vi "Fetch Multi Eval Meas List ACLR Detected Allocation Results.vi"(8 "error in (no error)":errorcluster, 10 "Instance (1)":T2=1, 11 "VISA resource name":refnum<visa-resource-name>) -> (0 "error out":errorcluster, 2 "Reliability":i32, 3 "VISA resource name out":refnum<visa-resource-name>)   [LabVIEW 2015, in "Rohde&Schwarz CMXP NR FR2 Measurement.lvlib"]
doc: "Returns the detected allocation for all measured list mode segments.\n\nAttribute:\nRSCMXPNRFR2M_ATTR_FETCH_MULTI_EVAL_MEASUREMENT_LIST_ACLR_DETECTED_ALLOCATION\n\nRemote-control command:\nFETCh:NRMMw:MEAS<i>:MEValuation:LIST:ACLR:DALLocation?"
uses:
  <instrlib>/Rohde&Schwarz CMXP NR FR2 Measurement/Rohde&Schwarz CMXP NR FR2 Measurement.lvlib
  <instrlib>/Rohde&Schwarz CMXP NR FR2 Measurement/Private/_Instance.ctl
panel:
  out "Detected Allocation Results":T1(array[cluster])
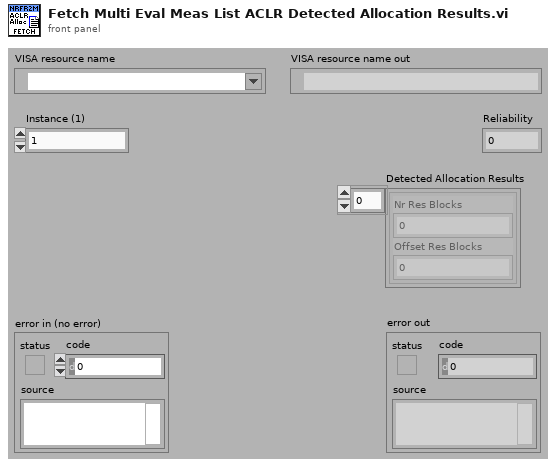
[diagram p1: front panel]
types:
  T1 = cluster{"Nr Res Blocks":i32, "Offset Res Blocks":i32}[]
  T2 = typedef "Rohde&Schwarz CMXP NR FR2 Measurement.lvlib/_Instance.ctl" = i32
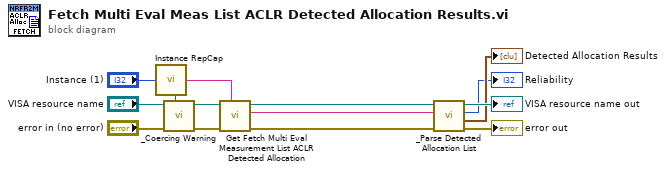
[diagram p0: block diagram]
diagram:
  n1 = call <instrlib>:"Instance RepCap.vi"("Instance In"="Instance (1)") -> ("In Range?"=w12:bool, "RepCap Identifier Out"=w4:string)  [unwired: 1 in]
  n2 = call <instrlib>:"_Coercing Warning.vi"("In Range?"=w12, "error in (no error)"="error in (no error)", "VISA resource name"="VISA resource name") -> ("error out"=w11:errorcluster, "VISA resource name out"=w10:refnum<visa-resource-name>)  [unwired: 7 in]
  n3 = call "Get Fetch Multi Eval Measurement List ACLR Detected Allocation"("Repeated Capabilities"=w4, "error in (no error)"=w11, "instrument handle"=w10) -> ("error out"=w7:errorcluster, "Fetch Multi Eval Measurement List ACLR Detected Allocation"=w8:string, "instrument handle out"=w9:refnum<visa-resource-name>)  [unwired: 6 in]
  n4 = call <instrlib>:"_Parse Detected Allocation List.vi"("error in (no error)"=w7, "Input String"=w8, "VISA resource name"=w9) -> ("error out"=→"error out":errorcluster, "Results"=→"Detected Allocation Results":T1, "Reliability"=→"Reliability":i32, "VISA resource name out"=→"VISA resource name out":refnum<visa-resource-name>)  [unwired: 5 in]
